vi "Clear_Info.vi"(8 "error in (no error)":errorcluster, 9 "index in":string, 10 "buildObject":T1) -> (0 "error out":errorcluster, 1 "index out":string, 2 "buildObject out":T1)   [LabVIEW 2020, in "IB_RegGroup.lvclass"]
uses:
  <vilib>/AppBuilder/IB_Classes/RegGroup/IB_RegGroup.lvclass
  <vilib>/AppBuilder/IB_Classes/RegGroup/IB_RegGroup.lvclass/IB_RegGroup.ctl
  <vilib>/AppBuilder/IB_RW_Project/IB_RW_Project_PropBag_Action.ctl
  <vilib>/AppBuilder/IB_Classes/RegData/IB_RegData.lvclass
  <resource>/Framework/Providers/API/ItemRef.ctl
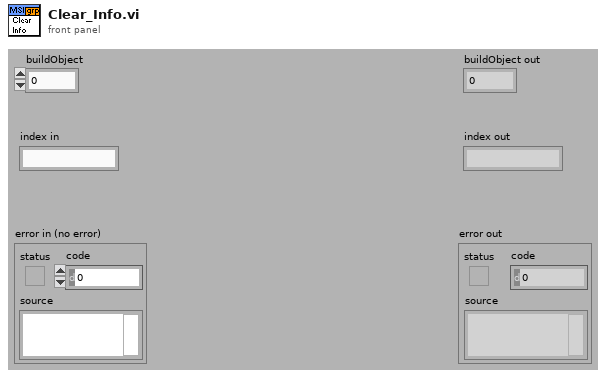
[diagram p1: front panel]
types:
  T1 = typedef "ItemRef.ctl" = u64
  T2 = typedef "IB_RW_Project_PropBag_Action.ctl" = enum16{"read", "write", "clear", "readPrevious", "writePrevious", "clearPrevious"}
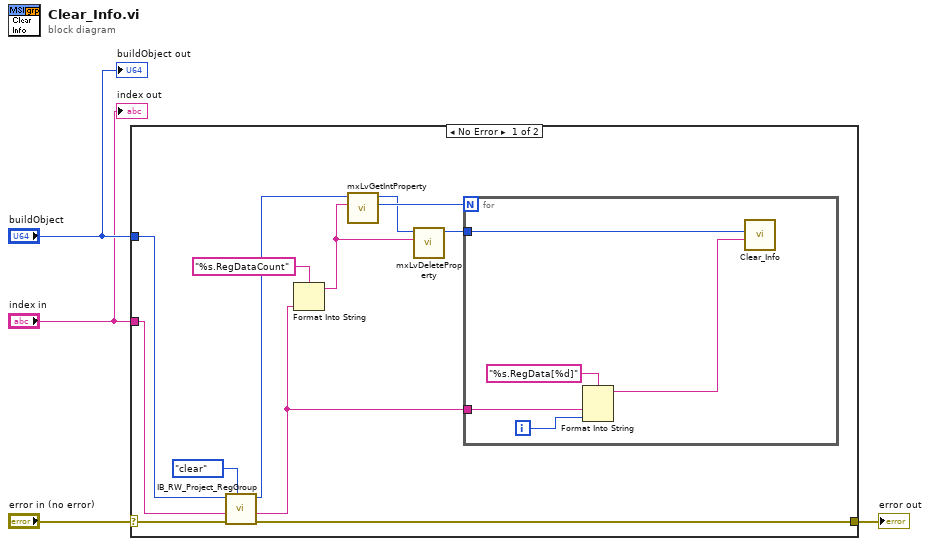
[diagram p0: block diagram]
diagram:
  n1 = case shown="No Error" "error in (no error)" {
    selector: "error in (no error)" -> [w14 w22]
    tunnel: [w13 w22] -> w3
    tunnel: "buildObject" -> [w11 _]
    tunnel: "index in" -> [w10 _]
    frame No Error {
      n2 = call <vilib>:"IB_RW_Project_RegGroup.vi"("action"=IB_RW_Project_PropBag_Action."clear", "error in (no error)"=w14, "index in"=w10, "buildObject"=w11) -> ("error out"=w13:errorcluster, "index out"=w9:string, "buildObject out"=w6:T1)  [unwired: 4 in, 1 out]
      n3 = Format Into String(format string="%s.RegDataCount", w9) -> (resulting string=w5:string)  [unwired: 2 in, 1 out]
      n4 = call <resource>:"mxLvGetIntProperty.vi"("Tag"=w5, "Item"=w6) -> ("Value"=w8:i32, "Item"=w7:T1)  [unwired: 1 in, 7 out]
      n5 = call <resource>:"mxLvDeleteProperty.vi"("Tag"=w5, "Item"=w7) -> ("Item"=w15:T1)  [unwired: 1 in, 8 out]
      n6 = for {
        N: w8 -> [_]
        tunnel: w15 -> [w21]
        tunnel: w9 -> [w18]
        i -> [w20]
        n7 = Format Into String(format string="%s.RegData[%d]", w18, w20) -> (resulting string=w17:string)  [unwired: 2 in, 1 out]
        n8 = call <vilib>:"Clear_Info.vi"("index in"=w17, "buildObject"=w21) -> ()  [unwired: 7 in, 3 out]
      }
    }
    frame Error {
    }
  }
  "error out" <- w3
  "index out" <- "index in"
  "buildObject out" <- "buildObject"
